vi "Goalie Normal.vi"(9 "balls":T1[](array[typedef]), 10 "Robot in":T3, 11 "IA State":T2={"our_robots"=[], "enemy_robots"=[], "balls"=[], "geometry"={"field_length"=0, "field_width"=0, "goal_width"=0, "goal_depth"=0, "center_circle_radius"=0, "defense_width"=0, "defense_depth"=0, "free_kick_from_defense_dist"=0, "penalty_spot_from_field_line_dist"=0, "penalty_line_from_spot_dist"=0, "half_moon_depth"=0, "half_moon_width"=0}, "IA Judge"={"stage"="", "command"="", "our_goalie_id"=0.0, "enemy_goalie_id"=0.0, "command enum"=enum."Halt", "Time"=enum."Azul"}, "Received Timestamp"=timestamp(0 s since 1904-01-01), "Events"={"Touch"=FALSE, "id touch"=0.0, "Ball out of \nVision"=FALSE, "Ball inside \nGoalie area"=FALSE, "Robot not responding"=FALSE, "Robots responding status"=[1.0, 1.0, 1.0, 1.0, 1.0, 1.0], "Enemy Ball \nPossession"=FALSE, "Id ini Possession"=0.0, "Ball Possesion"=FALSE, "Id Possesion"=0.0, "Ball at\nour goal side"=FALSE, "Ball at\ntouchline"=FALSE, "Ball at\nenemy goal side"=FALSE}}) -> (3 "Robot out":T3)   [LabVIEW 2018]
uses:
  Core/AI Robot.ctl
  Functions Enum.ctl
  AttackerStates.ctl
  Path Planning/RRT/PathDests.ctl
  Path Planning/RRT/PathDest.ctl
  Core/AI Input.ctl
  Core/AI Ball.ctl
  Core/Field Size.ctl
  Core/AI Judge.ctl
  Command Enum.ctl
  Util/Events/Events.ctl
  <vilib>/Analysis/_algsub.llb/Real Vector Norm.vi
  <vilib>/Analysis/NI_AALPro.lvlib
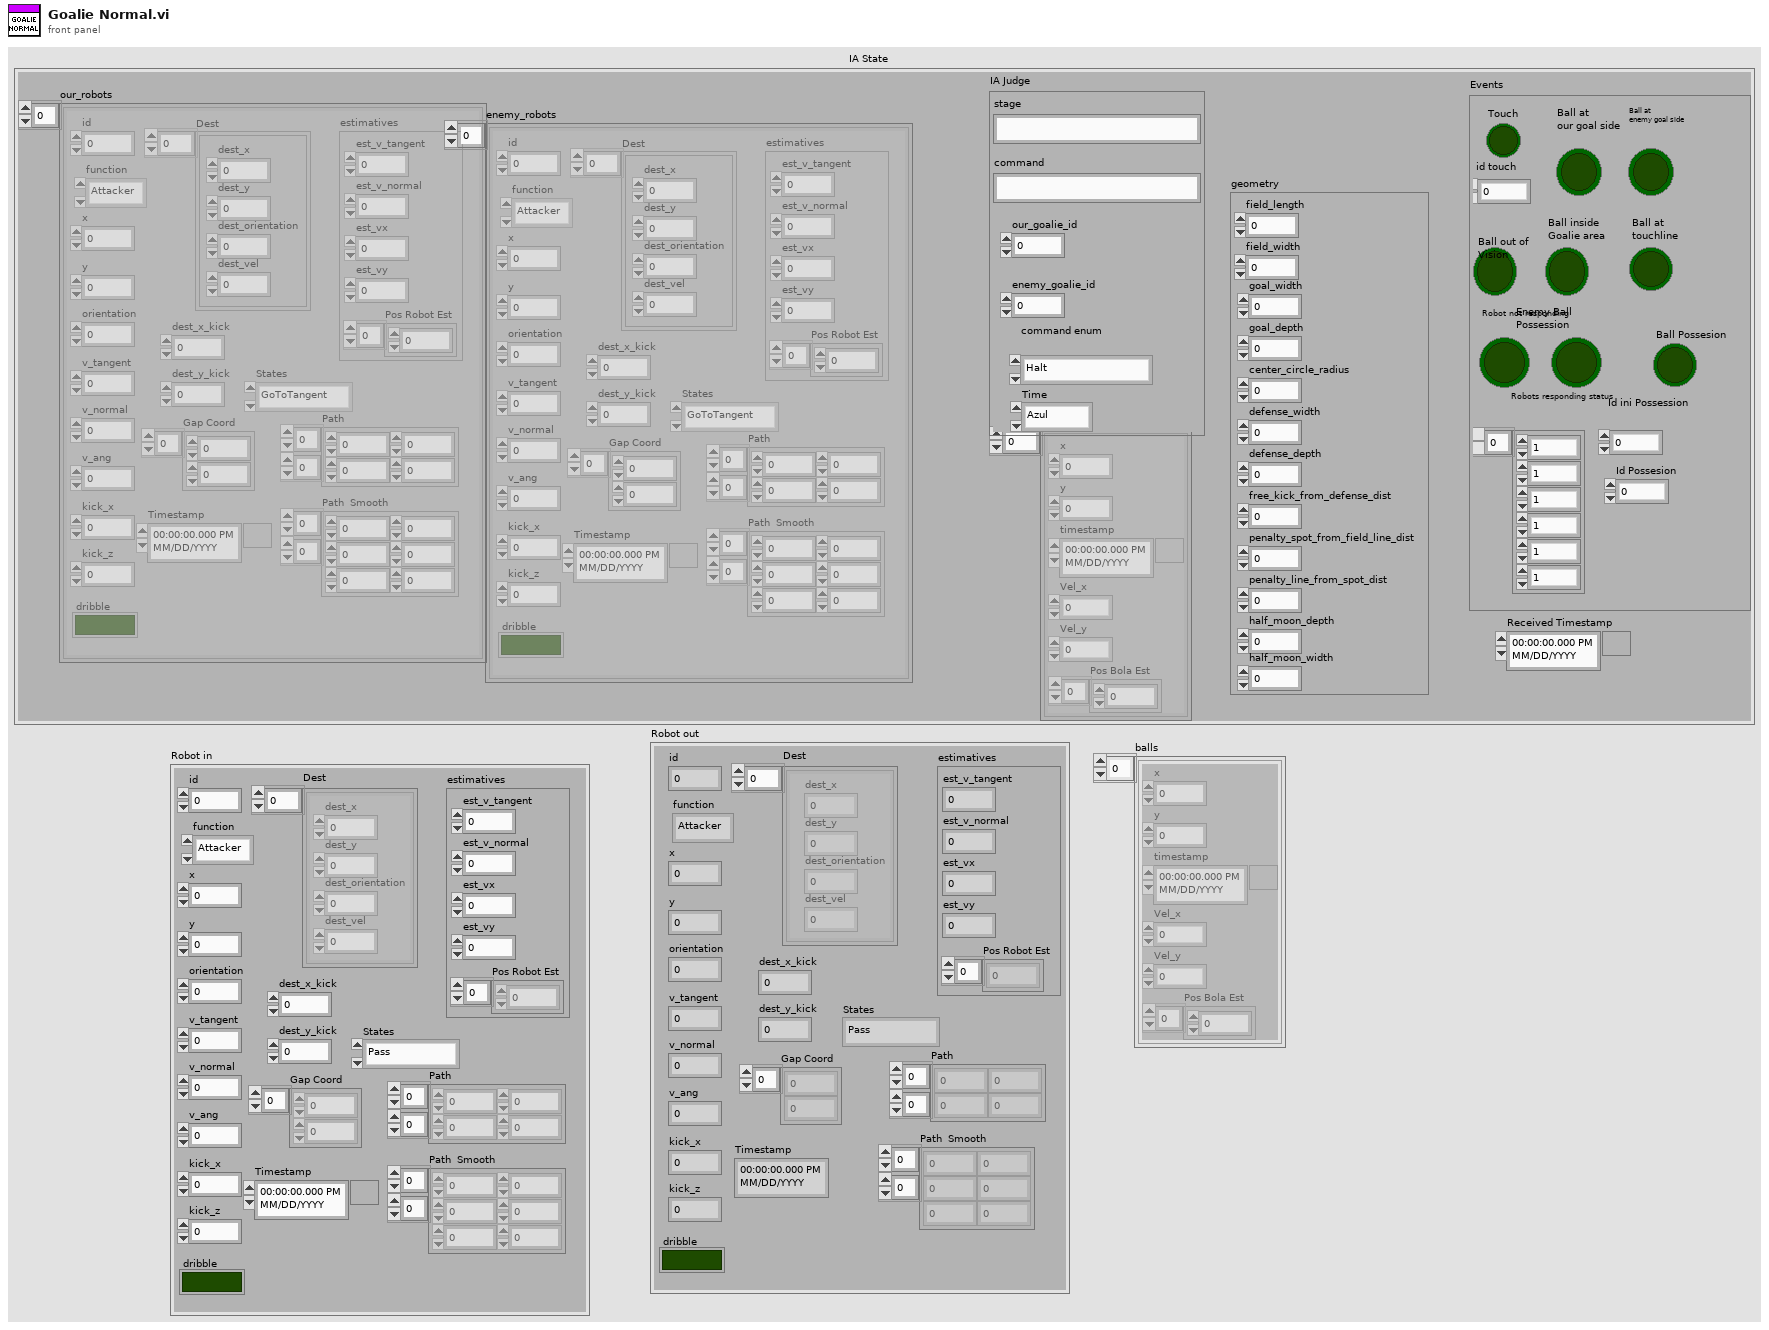
[diagram p1: front panel]
types:
  T1 = typedef "AI Ball.ctl" = cluster{"x":dbl, "y":dbl, "timestamp":timestamp, "Vel_x":dbl, "Vel_y":dbl, "Pos Bola Est":dbl[]}
  T2 = typedef "AI Input.ctl" = cluster{"our_robots":T3[], "enemy_robots":T3[], "balls":T1[], "geometry":T8, "IA Judge":T9, "Received Timestamp":timestamp, "Events":T11}
  T3 = typedef "AI Robot.ctl" = cluster{"id":u32, "function":T4, "x":dbl, "y":dbl, "orientation":dbl, "v_tangent":dbl, "v_normal":dbl, "v_ang":dbl, "kick_x":dbl, "kick_z":dbl, "dribble":bool, "Timestamp":timestamp, "estimatives":cluster{"est_v_tangent":dbl, "est_v_normal":dbl, "est_vx":dbl, "est_vy":dbl, "Pos Robot Est":dbl[]}, "dest_x_kick":dbl, "dest_y_kick":dbl, "Gap Coord":dbl[], "States":T5, "Path ":dbl[][], "Path  Smooth":dbl[][], "Dest":T6}
  T4 = typedef "Functions Enum.ctl" = enum16{"Attacker", "Goalie", "Defender", "Striker", "Goto 0", "Dummy", "Kicker", "ZigZag"}
  T5 = typedef "AttackerStates.ctl" = enum16{"Pass", "GoToTangent", "BallGetting", "GoToKick", "Rotate anti-clockwise", "Rotate Clockwise", ""}
  T6 = typedef "PathDests.ctl" = T7[]
  T7 = typedef "PathDest.ctl" = cluster{"dest_x":dbl, "dest_y":dbl, "dest_orientation":dbl, "dest_vel":dbl}
  T8 = typedef "Field Size.ctl" = cluster{"field_length":u32, "field_width":u32, "goal_width":u32, "goal_depth":u32, "center_circle_radius":u32, "defense_width":u32, "defense_depth":u32, "free_kick_from_defense_dist":u32, "penalty_spot_from_field_line_dist":u32, "penalty_line_from_spot_dist":u32, "half_moon_depth":u32, "half_moon_width":u32}
  T9 = typedef "AI Judge.ctl" = cluster{"stage":string, "command":string, "our_goalie_id":dbl, "enemy_goalie_id":dbl, "command enum":T10, "Time":enum16{"Azul", "Amarelo"}}
  T10 = typedef "Command Enum.ctl" = enum16{"Halt", "Stop", "Force Start", "PKA Normal Start", "Prepare Kickoff Ally", "PKE Normal Start", "Prepare Kickoff Enemy", "Prepare Penalty Ally", "PPA Normal Start", "Prepare Penalty Enemy", "PPE Normal Start", "Ball Placement Enemy Up", "Ball Placement Enemy Down", "Ball Placement Ally Up", "Ball Placement Ally Mid", "Ball Placement Ally Down", "Indirect Free Enemy", "Indirect Free Ally", "Timeout Enemy", "Timeout Ally", "Goal Enemy", "Goal Ally", "Normal Half Time", "Extra Time Break", "Extra Half Time", "None", "Post Game"}
  T11 = typedef "Events.ctl" = cluster{"Touch":bool, "id touch":dbl, "Ball out of \nVision":bool, "Ball inside \nGoalie area":bool, "Robot not responding":bool, "Robots responding status":dbl[], "Enemy Ball \nPossession":bool, "Id ini Possession":dbl, "Ball Possesion":bool, "Id Possesion":dbl, "Ball at\nour goal side":bool, "Ball at\ntouchline":bool, "Ball at\nenemy goal side":bool}
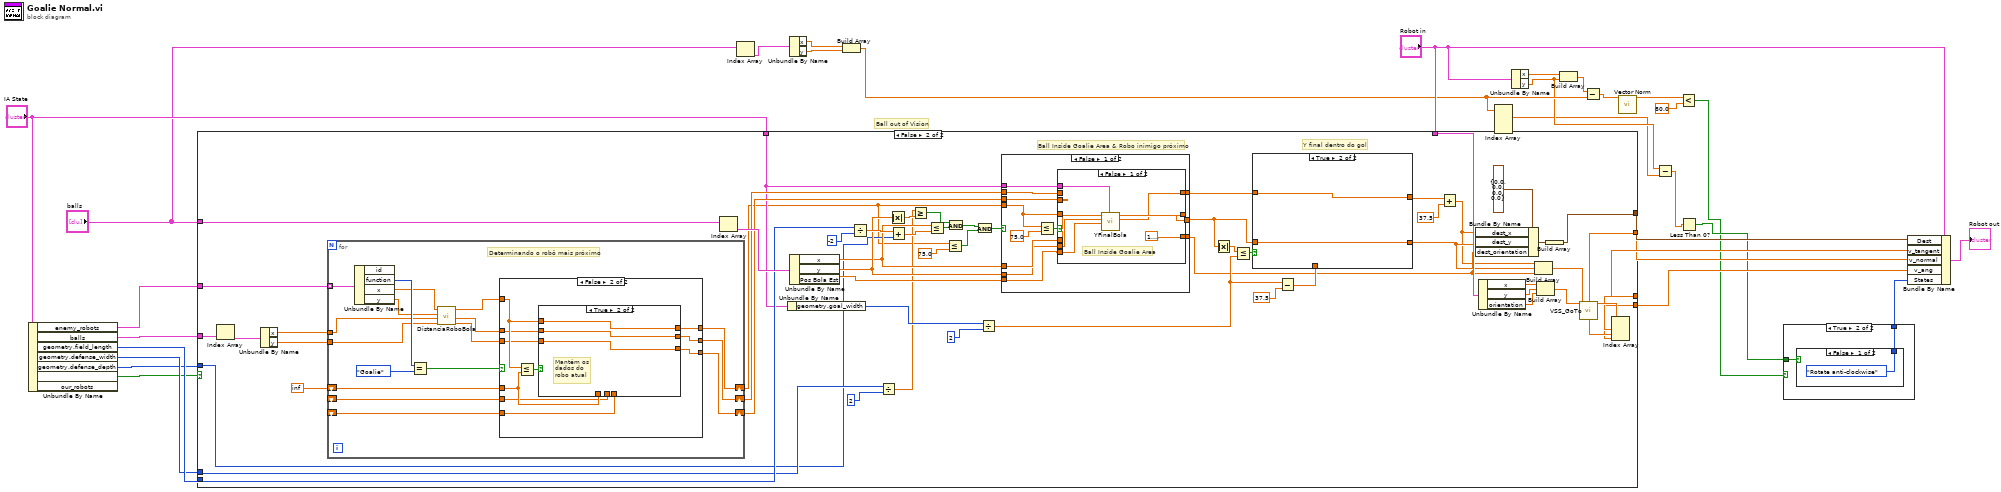
[diagram p0: block diagram]
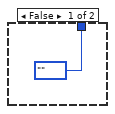
[diagram p2: hidden frame]
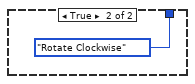
[diagram p3: hidden frame]
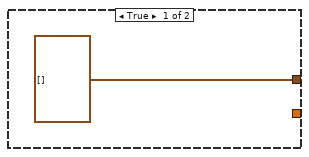
[diagram p4: hidden frame]
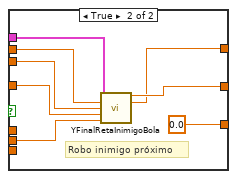
[diagram p5: hidden frame]
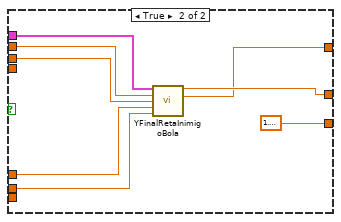
[diagram p6: hidden frame]
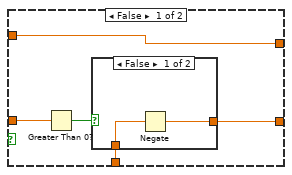
[diagram p7: hidden frame]
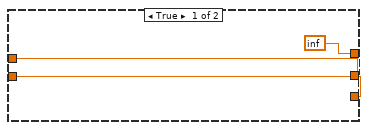
[diagram p9: hidden frame]
diagram:
  # "Ball out of Vision"
  n1 = Unbundle By Name("IA State") -> ("enemy_robots"=w26:T3[], "balls"=w27:T1[], "geometry.field_length"=w22:u32, "geometry.defense_width"=w20:u32, "geometry.defense_depth"=w19:u32, "Events.Ball out of \nVision"=w18:bool)  [unwired: 1 out]
  n2 = case shown="False" w18 {
    tunnel: [T7[] [] w87] -> w28
    tunnel: w27 -> [_ w83]
    tunnel: w26 -> [_ w82]
    tunnel: "balls" -> [_ w78]
    tunnel: "Robot in" -> [_ w70]
    tunnel: [_ w62] -> w25
    tunnel: [_ w61] -> w24
    tunnel: [_ w60] -> w23
    tunnel: w22 -> [_ w55]
    tunnel: "IA State" -> [_ w46]
    tunnel: w20 -> [_ w42]
    tunnel: w19 -> [_ w40]
    frame True {
    }
    frame False {
      # "Y final dentro do gol"
      # "Ball Inside Goalie Area & Robo inimigo próximo"
      n3 = Index Array(array=w83) -> (element=w84:T1)  [unwired: 1 in]
      n4 = Unbundle By Name(w84) -> ("x"=w81:dbl, "y"=w80:dbl)
      n5 = for {
        tunnel: w82 -> [w149] mode=indexing
        tunnel: w81 -> [w143]
        tunnel: w80 -> [w142]
        shift-right: [w136] -> w36
        shift-left: inf -> [w138]
        shift-right: [w134] -> w47
        shift-left: _ -> [w137]
        shift-right: [w133] -> w48
        shift-left: _ -> [w135]
        # "Determinando o robô mais próximo"
        n6 = Unbundle By Name(w149) -> ("function"=w147:T4, "x"=w145:dbl, "y"=w144:dbl)  [unwired: 1 out]
        n7 = Equal?(x=w147, y=Functions_Enum."Goalie") -> (x = y?=w146:bool)
        n8 = call "DistanciaRoboBola.vi"("Y bola"=w142, "X bola"=w143, "Y robo"=w144, "X robo"=w145) -> ("Y robo"=w139:dbl, "X robo"=w140:dbl, "Distância"=w141:dbl)  [unwired: 5 in]
        n9 = case shown="False" w146 {
          tunnel: w141 -> [_ w160]
          tunnel: w140 -> [w151 w159]
          tunnel: w139 -> [w150 w158]
          tunnel: w138 -> [_ w157]
          tunnel: w137 -> [_ w156]
          tunnel: [inf w162] -> w136
          tunnel: w135 -> [_ w153]
          tunnel: [w151 w155] -> w134
          tunnel: [w150 w154] -> w133
          frame True {
          }
          frame False {
            n10 = Less Or Equal?(x=w160, y=w157) -> (x <= y?=w161:bool)
            n11 = case shown="True" w161 {
              tunnel: [w164 w167] -> w155
              tunnel: [w165 w168] -> w162
              tunnel: w160 -> [_ w168]
              tunnel: w159 -> [_ w167]
              tunnel: w158 -> [_ w166]
              tunnel: w157 -> [w165 _]
              tunnel: w156 -> [w164 _]
              tunnel: w153 -> [w163 _]
              tunnel: [w163 w166] -> w154
              frame False {
                # "Mantém os\ndados do\nrobo anterior"
              }
              frame True {
                # "Mantém os\ndados do\nrobo atual"
              }
            }
          }
        }
      }
      n12 = Index Array(array=w78) -> (element=w77:T1)  [unwired: 1 in]
      n13 = Unbundle By Name(w46) -> ("geometry.goal_width"=w58:u32)
      n14 = Unbundle By Name(w77) -> ("x"=w49:dbl, "y"=w50:dbl, "Pos Bola Est"=w51:dbl[])
      n15 = Divide(x=w55, y=-2) -> (x/y=w54:dbl)
      n16 = Divide(x=w42, y=2) -> (x/y=w41:dbl)
      n17 = Absolute Value(x=w50) -> (abs(x)=w59:dbl)
      n18 = Add(x=w54, y=w40) -> (x+y=w53:dbl)
      n19 = Greater Or Equal?(x=w41, y=w59) -> (x >= y?=w57:bool)
      n20 = Less Or Equal?(x=w49, y=w53) -> (x <= y?=w52:bool)
      n21 = Less Or Equal?(x=w36, y=75.0) -> (x <= y?=w35:bool)
      n22 = And(x=w57, y=w52) -> (x .and. y?=w38:bool)
      n23 = And(x=w38, y=w35) -> (x .and. y?=w39:bool)
      n24 = Divide(x=w58, y=2) -> (x/y=w72:dbl)
      n25 = case shown="False" w39 {
        tunnel: w51 -> [w88 _]
        tunnel: w50 -> [w91 w118]
        tunnel: w49 -> [w92 w119]
        tunnel: w36 -> [w93 _]
        tunnel: w48 -> [w94 w120]
        tunnel: w47 -> [w95 w121]
        tunnel: w46 -> [w96 w122]
        tunnel: [w97 w116] -> w45
        tunnel: [w98 w117] -> w44
        tunnel: [w89 1.5707963267948966] -> w34
        frame False {
          n26 = Less Or Equal?(x=w93, y=75.0) -> (x <= y?=w90:bool)
          n27 = case shown="False" w90 {
            tunnel: w96 -> [w102 w113]
            tunnel: w95 -> [_ w112]
            tunnel: w94 -> [_ w111]
            tunnel: w92 -> [w106 _]
            tunnel: w91 -> [w105 w110]
            tunnel: [w104 w114] -> w98
            tunnel: w88 -> [w100 _]
            tunnel: [w103 w109] -> w97
            tunnel: w93 -> [_ w108]
            tunnel: [1.5707963267948966 0.0] -> w89
            frame False {
              # "Ball Inside Goalie Area"
              n28 = call "YFinalBola.vi"("IA State"=w102, "Pos Est"=w100, "Y bola"=w105, "X bola"=w106) -> ("X goleiro"=w103:dbl, "Y final da bola"=w104:dbl)  [unwired: 6 in]
            }
            frame True {
              # "Robo inimigo próximo"
              n29 = call "YFinalRetaInimigoBola.vi"("IA State"=w113, "X robo"=w112, "Y robo"=w111, "X bola"=w108, "Y bola"=w110) -> ("Y final da bola"=w114:dbl, "X goleiro"=w109:dbl)  [unwired: 9 in]
            }
          }
        }
        frame True {
          n30 = call "YFinalRetaInimigoBola.vi"("IA State"=w122, "X robo"=w121, "Y robo"=w120, "X bola"=w119, "Y bola"=w118) -> ("Y final da bola"=w117:dbl, "X goleiro"=w116:dbl)  [unwired: 9 in]
        }
      }
      n31 = Absolute Value(x=w44) -> (abs(x)=w76:dbl)
      n32 = Less Or Equal?(x=w76, y=w72) -> (x <= y?=w74:bool)
      n33 = Subtract(x=w72, y=37.5) -> (x-y=w71:dbl)
      n34 = case shown="True" w74 {
        tunnel: w44 -> [w127 w132]
        tunnel: [w124 w132] -> w65
        tunnel: [w123 w131] -> w33
        tunnel: w45 -> [w123 w131]
        tunnel: w71 -> [w125 _]
        frame False {
          n35 = Greater Than 0?(x=w127) -> (x > 0?=w126:bool)
          n36 = case shown="False" w126 {
            tunnel: [w128 w130] -> w124
            tunnel: w125 -> [w129 w130]
            frame False {
              n37 = Negate(x=w129) -> (-x=w128:dbl)
            }
            frame True {
            }
          }
        }
        frame True {
        }
      }
      n38 = Add(x=w33, y=37.5) -> (x+y=w31:dbl)
      n39 = Bundle By Name(cluster=T7 {"dest_x"=0.0, "dest_y"=0.0, "dest_orientation"=0.0, "dest_vel"=0.0} ("element"), "dest_x"=w31, "dest_y"=w65, "dest_orientation"=w34) -> (w86:T7)
      n40 = Unbundle By Name(w70) -> ("x"=w66:dbl, "y"=w69:dbl, "orientation"=w68:dbl)
      n41 = Build Array(w31, w65, w34) -> (w64:dbl[])
      n42 = Build Array(w66, w69, w68) -> (w67:dbl[])
      n43 = Build Array(w86) -> (w87:T7[])
      n44 = call "VSS_GoTo.vi"("SetPoint"=w64, "Position"=w67) -> ("Output Vel"=w63:dbl[])  [unwired: 9 in]
      n45 = Index Array(array=w63) -> (element #1=w62:dbl, element #2=w61:dbl, element #3=w60:dbl)  [unwired: 3 in]
    }
  }
  n46 = Index Array(array="balls") -> (element=w14:T1)  [unwired: 1 in]
  n47 = Unbundle By Name(w14) -> ("x"=w13:dbl, "y"=w12:dbl)
  n48 = Build Array(w13, w12) -> (w6:dbl[])
  n49 = Index Array(array=w6) -> (element #1=w3:dbl)  [unwired: 4 in, 3 out]
  n50 = Unbundle By Name("Robot in") -> ("x"=w16:dbl, "y"=w5:dbl)
  n51 = Build Array(w16, w5) -> (w11:dbl[])
  n52 = Subtract(x=w11, y=w6) -> (x-y=w9:dbl[])
  n53 = call-poly <vilib>:"Vector Norm.vi"("Input Vector"=w9) -> ("norm"=w8:dbl)  [unwired: 9 in, 1 out]
  n54 = Subtract(x=w5, y=w3) -> (x-y=w4:dbl)
  n55 = Less?(x=w8, y=80.0) -> (x < y?=w1:bool)
  n56 = Less Than 0?(x=w4) -> (x < 0?=w2:bool)
  n57 = case shown="True" w1 {
    tunnel: [AttackerStates."" ("States") w171] -> w7
    tunnel: w2 -> [_ w170]
    frame False {
    }
    frame True {
      n58 = case shown="False" w170 {
        tunnel: [AttackerStates."Rotate anti-clockwise" ("States") AttackerStates."Rotate Clockwise" ("States")] -> w171
        frame False {
        }
        frame True {
        }
      }
    }
  }
  n59 = Bundle By Name(cluster="Robot in", "Dest"=w28, "v_tangent"=w25, "v_normal"=w24, "v_ang"=w23, "States"=w7) -> (→"Robot out":T3)
